vi "Get Pin.vi"(0 "Arduino in":refnum<class "Arduino.lvclass">, 5 "VISA resource name":refnum<visa-resource-name>, 9 "Pin":dbl, 11 "error in (no error)":errorcluster) -> (4 "Arduino out":refnum<class "Arduino.lvclass">, 6 "VISA resource name 2":refnum<visa-resource-name>, 8 "Boolean":bool, 10 "Response":string, 15 "error out":errorcluster)   [LabVIEW 2020, in "Arduino.lvclass"]
uses:
  Arduino.lvclass
  Abstract/Serial Device/Serial Device.lvclass
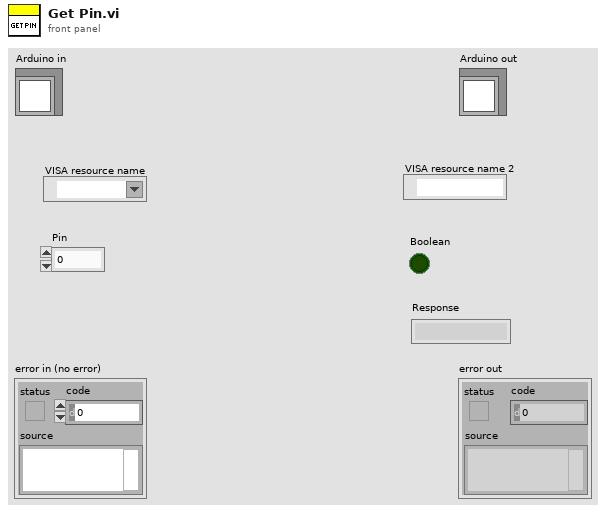
[diagram p1: front panel]
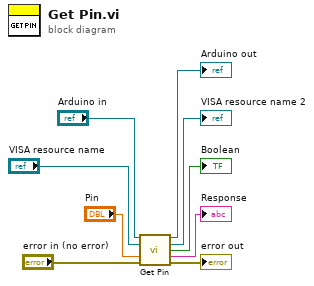
[diagram p0: block diagram]
diagram:
  n1 = call-parent "Get Pin.vi"("Serial Device in"="Arduino in", "VISA resource name"="VISA resource name", "Pin"="Pin", "error in (no error)"="error in (no error)") -> ("Serial Device out"=→"Arduino out":refnum<class "Arduino.lvclass">, "VISA resource name 2"=→"VISA resource name 2":refnum<visa-resource-name>, "Boolean"=→"Boolean":bool, "Response"=→"Response":string, "error out"=→"error out":errorcluster)  [unwired: 7 in]
